vi "chart series set trendline forecast.vi"(8 "error in (no error)":errorcluster, 9 "backward":dbl, 10 "forward":dbl, 11 "series":u32) -> (0 "error out":errorcluster)   [LabVIEW 8.6]
doc: "void chart_series_set_trendline_forecast(lxw_chart_series series, double forward, double backward);"
uses:
  pending_lvxlsxwriter/xlsxwriter.dll
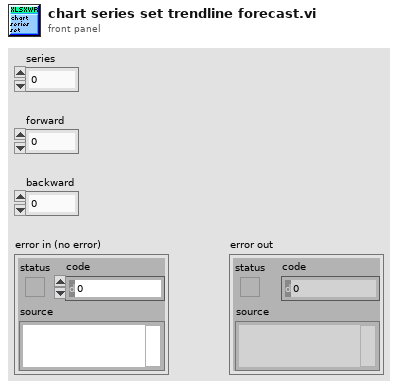
[diagram p1: front panel]
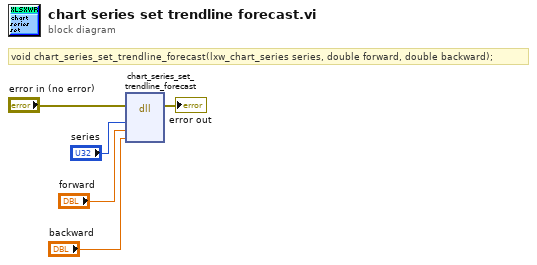
[diagram p0: block diagram]
diagram:
  # "void chart_series_set_trendline_forecast(lxw_chart_series series, double forward, double backward);"
  n1 = dll-call lib="C:/Users/WDAGUtilityAccount/Desktop/pending_lvxlsxwriter/xlsxwriter.*" fn="chart_series_set_trendline_forecast"(error in="error in (no error)", "series"="series", "forward"="forward", "backward"="backward") -> (error out=→"error out":errorcluster)  [unwired: 6 in, 1 out]
